vi "DAC text to num.vi"(11 "In Array":T2(array[cluster])) -> (3 "Out Array":T1(array[cluster]))   [LabVIEW 2017]
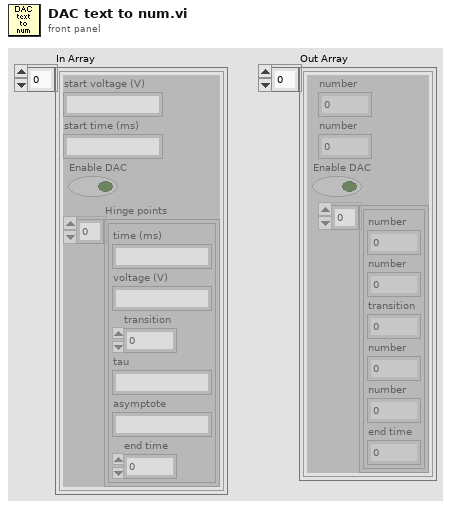
[diagram p1: front panel]
types:
  T1 = cluster{"number":dbl, "number":dbl, "Enable DAC":bool, cluster{"number":dbl, "number":dbl, "transition":u16, "number":dbl, "number":dbl, "end time":dbl}[]}[]
  T2 = cluster{"start voltage (V)":string, "start time (ms)":string, "Enable DAC":bool, "Hinge points":cluster{"time (ms)":string, "voltage (V)":string, "transition":u16, "tau":string, "asymptote":string, "end time":dbl}[]}[]
  T3 = cluster{"time (ms)":string, "voltage (V)":string, "transition":u16, "tau":string, "asymptote":string, "end time":dbl}[]
  T4 = cluster{"number":dbl, "number":dbl, "transition":u16, "number":dbl, "number":dbl, "end time":dbl}
  T5 = cluster{"number":dbl, "number":dbl, "Enable DAC":bool, cluster{"number":dbl, "number":dbl, "transition":u16, "number":dbl, "number":dbl, "end time":dbl}[]}
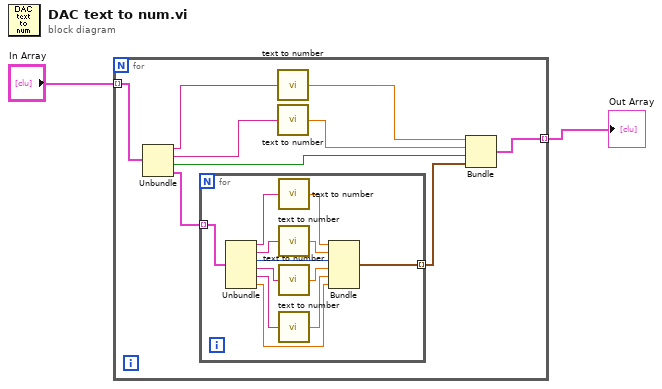
[diagram p0: block diagram]
diagram:
  n1 = for {
    tunnel: "In Array" -> [w11] mode=indexing
    tunnel: [w3] -> w1 mode=indexing
    n2 = Unbundle(w11) -> ("start voltage (V)"=w9:string, "start time (ms)"=w7:string, "Enable DAC"=w5:bool, "Hinge points"=w10:T3)
    n3 = for {
      tunnel: w10 -> [w23] mode=indexing
      tunnel: [w12] -> w4 mode=indexing
      n4 = Unbundle(w23) -> ("time (ms)"=w22:string, "voltage (V)"=w21:string, "transition"=w16:u16, "tau"=w20:string, "asymptote"=w19:string, "end time"=w13:dbl)
      n5 = call "text to number.vi"("text"=w22) -> ("number"=w18:dbl)
      n6 = call "text to number.vi"("text"=w21) -> ("number"=w17:dbl)
      n7 = call "text to number.vi"("text"=w20) -> ("number"=w15:dbl)
      n8 = call "text to number.vi"("text"=w19) -> ("number"=w14:dbl)
      n9 = Bundle("number"=w18, "number"=w17, "transition"=w16, "number"=w15, "number"=w14, "end time"=w13) -> (w12:T4)  [unwired: 1 in]
    }
    n10 = call "text to number.vi"("text"=w9) -> ("number"=w8:dbl)
    n11 = call "text to number.vi"("text"=w7) -> ("number"=w6:dbl)
    n12 = Bundle("number"=w8, "number"=w6, "Enable DAC"=w5, w4) -> (w3:T5)  [unwired: 1 in]
  }
  "Out Array" <- w1
